vi "Stop Motor.vi"(9 "Message handler data":T1) -> ()   [LabVIEW 2018]
uses:
  Type Defs/Message loop data.ctl
  Type Defs/FPGA reference.ctl
  Type Defs/RT Status.ctl
  <vilib>/Utility/error.llb/Error Cluster From Error Code.vi
  <vilib>/rvi/errors/niLvFpgaAdjustHostInterfaceError.vi
  <vilib>/rvi/interface/nirviReadWriteControl/nirviReadWriteControl.xnode
  FPGA Bitfiles/CompressorRigV2_CompressorFPGA_FPGAMainV3_7sPRekuravM.lvbitx
  NiFpgaLv.dll
types:
  T1 = typedef "Message loop data.ctl" = cluster{"Parameters":cluster{"FPGA Ref":T2, "configID":u32, "activeChannels":cluster{"index":u16, "name":string}[]}, "Variables":cluster{"RT Status":T3, "watchdog":timestamp, "limitsEnabled":bool, "Interlocks":cluster{"gearboxOil":bool, "bearingOil":bool, "gearboxAir":bool}}}
  T2 = typedef "FPGA reference.ctl" = refnum<k20>
  T3 = typedef "RT Status.ctl" = cluster{"Comms loop":bool, "scheduler loop":bool, "data process loop":bool, "FIFO loop":bool, "Command Stream":bool, "Error Stream":bool, "FPGA FIFO":bool, "Data Stream":bool}
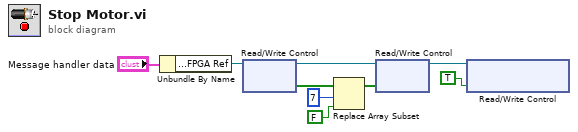
[diagram p0: block diagram]
diagram:
  n1 = Unbundle By Name("Message handler data") -> ("Parameters.FPGA Ref"=w8:T2)
  n2 = xnode "Read/Write Control"("FPGA VI Reference In"=w8) -> ("FPGA VI Reference Out"=w5:T2, "Mod 8"=w4:bool[])  [unwired: 1 in, 1 out]
  n3 = Replace Array Subset(array=w4, new element=FALSE ("new element/subarray"), index=7) -> (w3:bool[])
  n4 = xnode "Read/Write Control"("FPGA VI Reference In"=w5, "Mod 8"=w3) -> ("FPGA VI Reference Out"=w7:T2)  [unwired: 1 in, 1 out]
  n5 = xnode "Read/Write Control"("FPGA VI Reference In"=w7, "Update Outputs"=TRUE ("Enable Data FIFO")) -> ()  [unwired: 1 in, 2 out]
